vi "Example Usage.vi"() -> ()   [LabVIEW 2013, in "Robust CSV.lvlib"]
uses:
  Robust CSV.lvlib
  Write CSV File_2D.vi
panel:
  out "CSV Data":string[][](array[string])
  out "error out":errorcluster
  # "Press run and open \"MOCK_DATA.csv\" then save to \"MOCK_DATA_new.csv\"\nThe interpreted data from \"MOCK_DATA.csv\" is displayed above."
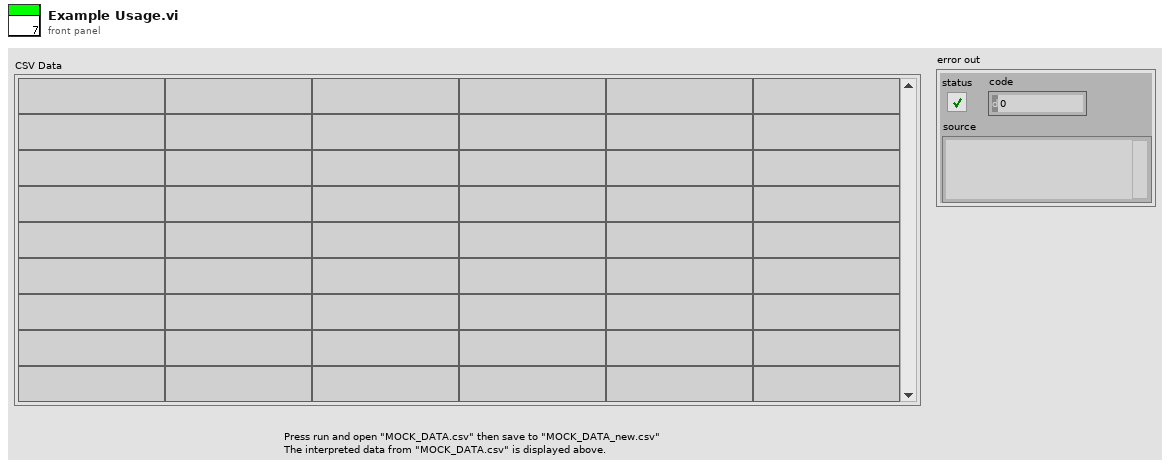
[diagram p1: front panel]
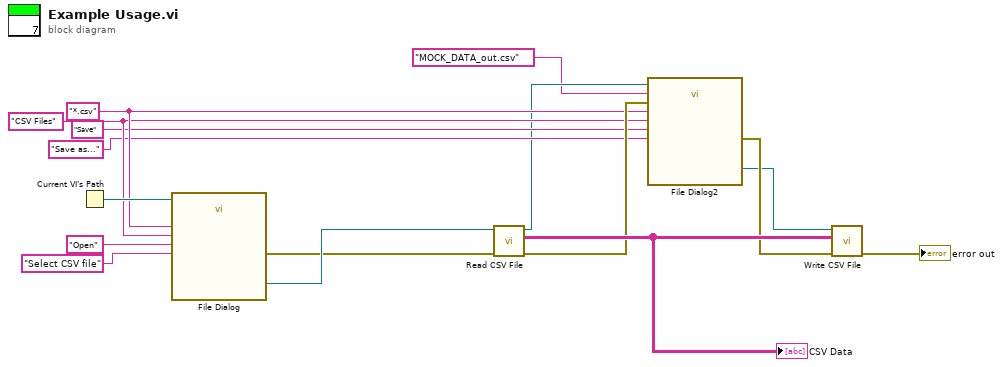
[diagram p0: block diagram]
diagram:
  w6 = "CSV Files" ("pattern label")
  w7 = "*.csv" ("pattern (all files)")
  n1 = Current VI's Path() -> (path=w11:path)
  n2 = call "File Dialog"("start path"=w11, "prompt"="Select CSV file", "button label"="Open", "pattern (all files)"=w7, "pattern label"=w6) -> ("selected path"=w14:path, "error out"=w13:errorcluster)  [unwired: 7 in, 2 out]
  n3 = call "Read CSV File.vi"("error in (no error)"=w13, "file path in"=w14) -> ("error out"=w10:errorcluster, "2-D array"=w16:string[][], "file path out"=w2:path)  [unwired: 7 in]
  "CSV Data" <- w16
  n4 = call "File Dialog2"("start path"=w2, "prompt"="Save as...", "button label"="Save", "default name"="MOCK_DATA_out.csv", "error in"=w10, "pattern (all files)"=w7, "pattern label"=w6) -> ("selected path"=w8:path, "error out"=w9:errorcluster)  [unwired: 5 in, 2 out]
  n5 = call-poly "Write CSV File.vi"("error in (no error)"=w9, "2D array"=w16, "file path in"=w8) -> ("error out"=→"error out":errorcluster)  [unwired: 7 in, 1 out]
